vi "Read Control Label.vi"(8 "error in (no error)":errorcluster, 11 "TreeItemCloseMsg in":refnum<class "TreeItemCloseMsg.lvclass">) -> (0 "error out":errorcluster, 2 "Control Label":string, 3 "TreeItemCloseMsg out":refnum<class "TreeItemCloseMsg.lvclass">)   [LabVIEW 2018, in "MVA Framework.lvlib" / "ActorEvents.lvlib" / "TreeItemCloseMsg.lvclass"]
uses:
  TreeItemCloseMsg.lvclass
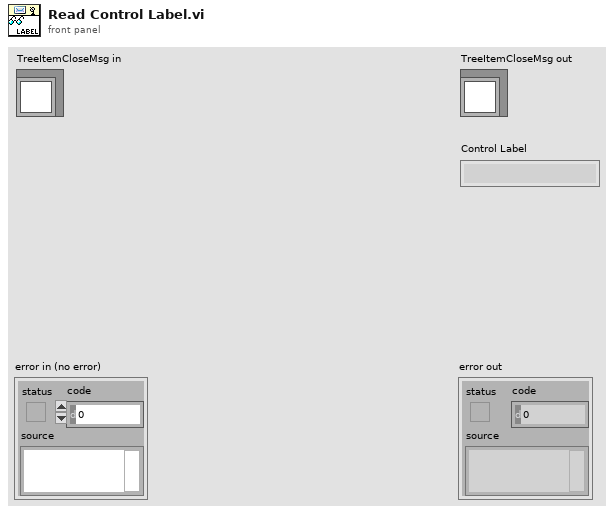
[diagram p1: front panel]
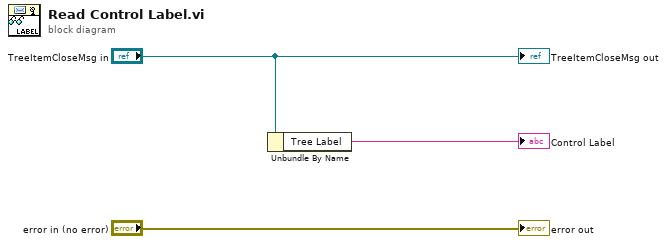
[diagram p0: block diagram]
diagram:
  n1 = Unbundle By Name("TreeItemCloseMsg in") -> ("Tree Label"=→"Control Label":string)
  "error out" <- "error in (no error)"
  "TreeItemCloseMsg out" <- "TreeItemCloseMsg in"
